vi "DtOLCloseTask.vi"(8 "Error in":errorcluster, 11 "Task in":i32) -> (0 "Error Out":errorcluster)   [LabVIEW 2016]
doc: "Stops the task if it is running and releases all resources that are associated with the task. After a task is closed, you can no longer use it."
uses:
  <userlib>/LV-Link3/DtLvLink.lvlib
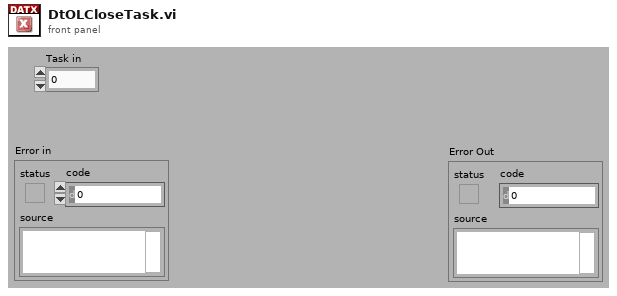
[diagram p1: front panel]
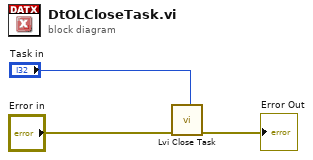
[diagram p0: block diagram]
diagram:
  n1 = call <userlib>:"Lvi Close Task.vi"("error in (no error)"="Error in", "TaskRef"="Task in") -> ("error out"=→"Error Out":errorcluster)  [unwired: 8 in, 1 out]
